vi "Read Parameter from Word.vi"(8 "error in":errorcluster, 9 "parameter definition":T1={"start index"=10, "size"=19, "encoding"=enum."BNR", "signed"=FALSE, "scale multiplier"=1.0, "scale offset"=0.0}, 11 "32-bit Word in":refnum<class "32-bit Word.lvclass">) -> (0 "error out":errorcluster, 2 "parameter value":dbl, 3 "32-bit Word out":refnum<class "32-bit Word.lvclass">)   [LabVIEW 2020, in "32-bit Word.lvclass"]
uses:
  32-bit Word.lvclass
  Parameter Definition.ctl
  <vilib>/NI/NI VeriStand Encoding and Decoding/Encoding.ctl
  32-bit Word.lvclass/32-bit Word.ctl
  Read 32-Bit Word.vi
  ARINC 429.lvclass
  <vilib>/NI/NI VeriStand Encoding and Decoding/Encoding and Decoding.lvlib
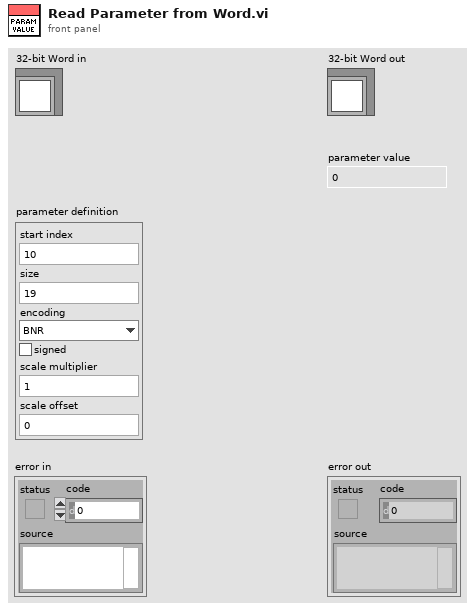
[diagram p1: front panel]
types:
  T1 = typedef "ARINC 429.lvclass/Parameter Definition.ctl" = cluster{"start index":i32, "size":i32, "encoding":T2, "signed":bool, "scale multiplier":dbl, "scale offset":dbl}
  T2 = typedef "Encoding and Decoding.lvlib/Encoding.ctl" = enum16{"BNR", "BCD", "Discrete"}
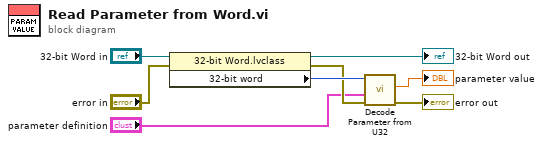
[diagram p0: block diagram]
diagram:
  n1 = property on="Property Node" class="32-bit Word.lvclass"(reference="32-bit Word in", error in="error in") -> (reference out=→"32-bit Word out":refnum<class "32-bit Word.lvclass">, error out=w4:errorcluster, "32-bit word"=w8:u32)
  n2 = call "Decode Parameter from U32.vi"("error in"=w4, "parameter definition"="parameter definition", "32-bit word in"=w8) -> ("error out"=→"error out":errorcluster, "value"=→"parameter value":dbl)  [unwired: 6 in, 1 out]
